vi "SENS_MULT_TSET_PORT_S_A_B.vi"(0 "VISA IN":refnum<visa-resource-name>, 1 "ID":i32, 2 "Output Port":string, 5 "error in":errorcluster, 7 "Channel":i32) -> (14 "VISA Out":refnum<visa-resource-name>, 19 "error out":errorcluster)   [LabVIEW 2018, in "PNA-X.lvlib"]
doc: "SENSe<cnum>:MULTiplexer<id>:TSET9:PORT3 <char> Superseded \nNote: This command is replaced with SENS:MULT:ALLPorts which sets ALL ports to the specified \noutputs. \n(Read-Write) Switches Port 3 of the specified E5091A to one of the available outputs. \nParameters \n<cnum> Any existing channel number; if unspecified, value is set to 1. \n<id> Id of the E5091A test set. Choose from 1 or 2. Learn how to set ID value. \n<char> Output port to be switched to. Choose from: \nR1 (R1+) \nR2 (R2+) \n1787\n\nR3 (R3+) If option 007 (7port), R2 is selected. \nExamples SENS:MULT1:TSET9:PORT3 R2 \nQuery Syntax SENSe<cnum>:MULTiplexer<id>:TSET9:PORT3? \nReturn Type Character \nDefault R1"
uses:
  PNA-X.lvlib
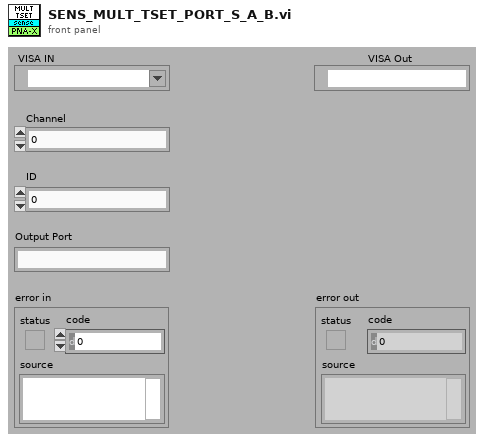
[diagram p1: front panel]
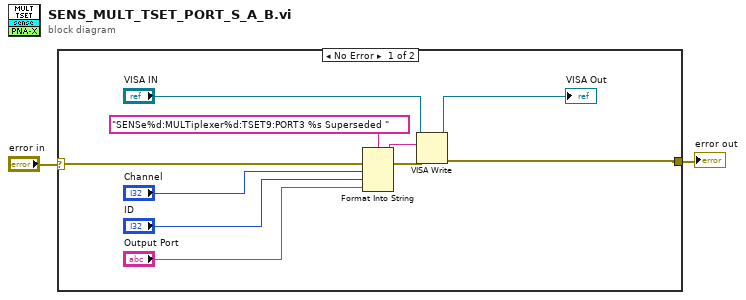
[diagram p0: block diagram]
diagram:
  n1 = case shown="No Error" "error in" {
    selector: "error in" -> [w12 w13]
    tunnel: [w7 w13] -> w1
    frame No Error {
      n2 = Format Into String(format string="SENSe%d:MULTiplexer%d:TSET9:PORT3 %s Superseded " ("Cmdline"), error in=w12, "Channel", "ID", "Output Port") -> (resulting string=w10:string, error out=w11:errorcluster)  [unwired: 1 in]
      n3 = VISA Write(VISA resource name="VISA IN", write buffer=w10, error in (no error)=w11) -> (VISA resource name out=→"VISA Out":refnum<visa-resource-name>, error out=w7:errorcluster)  [unwired: 1 out]
    }
    frame Error {
    }
  }
  "error out" <- w1
